vi "GetWindowFromID.vi"(8 "No Error":errorcluster, 11 "WindowID":T1) -> (0 "Error Out":errorcluster, 3 "Window [SDL_Window *]":T2 format="%.0x")   [LabVIEW 2026, in "SDL3.lvlib" / "Video.lvlib"]
doc: "<B>Summary</B>\nGet a window from a stored ID.\n\n<B>Remarks</B>\nThe numeric ID is what SDL_WindowEvent references, and is necessary to map these events to specific SDL_Window objects."
uses:
  Video.lvlib
  WindowID--integer.ctl
  <vilib>/Utility/error.llb/Error Cluster From Error Code.vi
  Error/Error.lvlib
  Lib/SDL3.dll
  SDL_Window--pointer.ctl
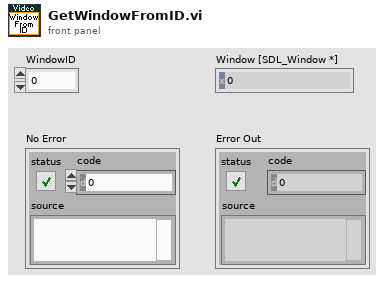
[diagram p1: front panel]
types:
  T1 = typedef "SDL3.lvlib/Video.lvlib/WindowID--integer.ctl" = u32
  T2 = typedef "SDL3.lvlib/Video.lvlib/SDL_Window--pointer.ctl" = i64
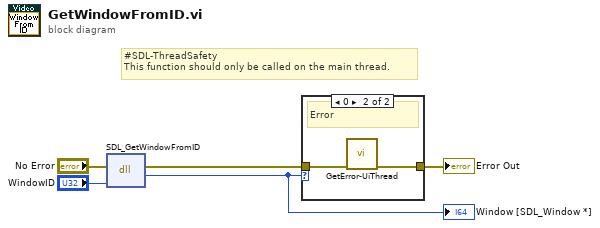
[diagram p0: block diagram]
diagram:
  # "#SDL-ThreadSafety\nThis function should only be called on the main thread."
  n1 = dll-call lib="C:/Users/saukko/Dev/LV-SDL3/Sources/SDL3/Lib/SDL3.*" fn="SDL_GetWindowFromID"(error in="No Error", "id"="WindowID") -> (error out=w1:errorcluster, "return type"=w4:i64)  [unwired: 3 in, 1 out]
  "Window [SDL_Window *]" <- w4
  n2 = case shown="0" w4 {
    tunnel: w1 -> [w6 w8]
    tunnel: [w6 w7] -> w2
    frame Default {
      # "Ok"
    }
    frame 0 {
      # "Error"
      n3 = call "GetError-UiThread.vi"("No Error"=w8) -> ("error out"=w7:errorcluster)  [unwired: 10 in]
    }
  }
  "Error Out" <- w2
